vi "Post-Processing VI Bin Files SubSample Tianyi.vi"() -> ()   [LabVIEW 2014]
uses:
  <vilib>/Utility/config.llb/NI_LVConfig.lvlib
  <vilib>/Utility/config.llb/Read Key (I32).vi
  <vilib>/Utility/config.llb/Read Key (Double).vi
  Classes/Processing/Processing.lvclass
panel:
  in  "A-Scan Change":i32=627
  out "BScan":u8[][](graph)
  out "Range":dbl=4.0
  out "Bits":dbl=16.0
  out "Points Per A Scan":i32=1600
  out "A-Scans Per BScan":i32=1000
  in  "Min / Max in dB (Contrast)":cluster{dbl, dbl}(slide)={-34.05144694533762, 14.823151125401928} scale=-40.0..60.0
  in  "Create 3D Data":bool=TRUE
  in  "Max":sgl=14.823152 format="%0.2f"
  in  "Min":sgl=-34.05145 format="%0.2f"
  out "Binary File Handle":refnum<file>
  in  "Create En Face Software Event":bool=TRUE
  out "En Face":sgl[][](graph)=[[-7.930091, -7.8040323, -7.973442, -8.000936, -7.8626037, -7.893125, -7.976362, -7.866958, -7.8874545, -8.053767, -7.895429, -8.001336, -8.058077, -7.9112062, -7.757364, -7.965038, -7.9575043, -8.167074, -8.054711, -8.167959, -7.8551683, -7.915979, -7.9114604, -7.864061, -8.055119, -7.9877367, -8.029805, -7.988413, -8.037094, -7.922483, -8.156847, -7.9672847, -7.8064103, -7.9114566, -7.773133, -7.9002914, -8.085471, -7.9221673, -7.957444, -7.958286, -7.698463, -8.002342, -7.989561, -7.952671, -7.984078, -7.836235, -8.0634165, -8.028308, -8.039231, -8.056543, -7.8877096, -7.9473996, -7.865986, -7.929803, -7.9396944, -7.8729186, -7.962053, -7.976538, -7.829268, -7.759593, -7.6770754, -7.917806, -7.978408, -7.7964263, -7.9014854, -7.8359327, -8.019228, -7.9651647, -7.961875, -8.0167675, -7.915086, -7.975068, -8.046566, -7.960596, -7.990237, -8.160412, -8.09407, -7.795923, -7.8977365, -7.917423, -8.06519, -7.941408, -8.036876, -7.946509, -8.009643, -7.7677317, -8.056414, -8.105821, -8.020063, -7.946077, -7.9010644, -8.056617, -8.010448, -8.0648775, -7.9236917, -7.8220835, -7.8197546, -7.8338175, -7.908895, -7.9036684, -7.9667068, -8.103706, -7.9954534, -7.9504957, -7.829475, -7.831149, -8.244316, -8.030985, -8.157568, -7.6754923, -7.9325967, -8.037667, -7.9114547, -7.946226, -7.8830395, -7.788606, -8.123245, -7.848808, -8.020647, -7.825039, -8.136002, -7.8881106, -7.840354, -7.8498588, -7.868983, -8.012706, -8.025735, -8.1118145, -7.816016, -7.8430986, -7.9750667, -8.042043, -7.820652, -7.8192554, -7.888372, -8.02898, -7.891756, -7.86369, -7.979582, -7.7987456, -8.169637, -7.8604546, -8.097469, -7.882909, -7.745224, -7.9409885, -8.008719, -7.874554, -7.934384, -7.889922, -7.9307194, -7.976539, -7.8116565, -8.037268, -7.8819757, -7.90127, -8.004612, -7.9514766, -7.6461873, -8.051855, -8.033362, -7.820009, -8.007025, -7.9113975, -7.972308, -8.075444, -7.9308887, -8.089264, -7.8016825, -7.919436, -7.94926, -7.7312274, -8.1581135, -7.806207, -7.956523, -7.9414477, -7.9876857, -7.9657526, -7.8116117, -7.8548036, -7.9839373, -7.9158034, -7.898539, -7.780124, -7.9533, -7.8764243, -7.739191, -7.80521, -8.063391, -7.9777446, -7.7854123, -7.9521074, -7.98957, -7.888753, -7.7991505, -7.9267855, -7.9612865, -7.819488, -7.865055, -8.14359, -7.7728977, -8.085733, -7.8384624, -7.743552, -7.886237, -7.9267993, -7.9535413, -7.8223243, -7.8396297, -7.870655, -8.026216, -7.7772164, -7.80645, -8.013777, -8.012371, -7.7353735, -7.935509, -7.860224, -7.9132657, -7.845752, -7.7870827, -7.958748, -8.160488, -7.869349, -7.78722, -7.955144, -7.8493533, -7.8096776, -7.986651, -7.945869, -7.935255, -8.144389, -7.9736667, -7.752922, -7.9255905, -7.974105, -7.799902, -7.6951523, -7.799085, -7.9162817, -8.017551, -7.9524965, -7.9512806, -8.165993, -7.7668185, -8.012505, -8.16206, -8.251981, -8.013035, -7.735666, -8.077859, -8.10991, -7.949526, -7.707088, -7.949591, -7.8823195, -7.816381, -8.034339, -7.868784, -7.89056, -7.8687153, -8.057175, -7.9518924, -7.9154468, -7.939955, -7.814576, -8.049959, -7.9097743, -7.863441, -7.846818, -7.96588, -7.789853, -8.094775, -7.7202816, -8.046873, -8.085813, -7.9780364, -7.9041257, -7.926487, -7.9343805, -8.040627, -7.830686, -8.070694, -7.8358226, -7.7780213, -7.8480616, -8.064976, -8.037013, -7.7728744, -8.012946, -7.9755006, -7.906261, -8.043798, -7.911961, -7.992775, -8.001271, -7.9195423, -8.082046, -8.020159, -7.9112606, -7.775108, -8.003549, -7.9803247, -7.8879714, -8.073655, -7.8865504, -7.783486, -7.8546762, -8.020269, -8.023449, -8.067884, -7.7598515, -7.90917, -8.069023, -7.7864647, -7.870191, -7.870761, -7.9444532, -7.993182, -7.917858, -8.03805, -7.93978, -7.7982545, -7.974645, -8.004379, -7.993704, -7.819672, -8.089255, -7.9242916, -7.907874, -7.9370337, -7.863256, -7.7989616, -7.80284, -8.006147, -7.823976, -7.995604, -8.050512, -7.964656, -8.11802, -7.9949827, -7.951066, -7.7912025, -7.927686, -8.008126, -7.891107, -8.10944, -8.134752, -7.8064127, -7.910995, -8.09849, -7.8788795, -8.016058, -7.8636923, -7.9307437, -7.974993, -7.991549, -7.974662, -7.93784, -7.7311897, -8.182317, -7.7587895, -8.095182, -7.874478, -7.813459, -7.879261, -7.829288, -8.035134, -7.861396, -7.986878, -7.782207, -7.79948, -7.9310637, -7.852276, -7.9916263, -7.9213424, -8.203527, -7.921085, -8.025147, -7.8967156, -7.8208995, -7.9961405, -8.083003, -7.98257, -7.9804964, -7.8674, -8.060883, -7.9558725, -7.945471, -8.142715, -8.087639, -8.218578, -8.243896, -7.959839, -7.9356184, -7.7503934, -8.0898695, -7.868658, -7.692663, -7.887905, -7.8621182, -7.9225054, -7.836562, -8.054047, -7.982782, -7.744281, -7.963519, -8.0447, -7.849429, -7.838456, -8.119481, -7.7900977, -7.9761267, -7.8695583, -7.76462, -7.970638, -7.9605556, -7.964503, -7.9509263, -7.86703, -8.055239, -7.884155, -7.844713, -7.856759, -7.9913874, -8.0371475, -7.938692, -8.049144, -8.021844, -7.7414804, -7.920646, -8.197608, -7.880194, -7.9744005, -8.035382, -8.069501, -8.181021, -8.0188465, -8.004074, -8.031586, -8.0189085, -8.058473, -7.9364552, -7.719303, -7.905371, -7.790757, -8.214631, -7.9018154, -7.987326, -7.9526286, -7.8612223, -7.9100804, -8.08193, -7.9836636, -8.027385, -8.095275, -7.9418774, -7.9966297, -7.9296713, -8.01897, -7.9224367, -7.8740377, -7.8067255, -8.113648, -7.965984, -7.919392, -7.9538283, -7.9669385, -7.9489245, -7.9807835, -8.049196, -8.2190485, -7.967722, -8.009465, -7.814837, -7.9246864, -7.923164, -7.990351, -7.917373, -8.095252, -8.055175, -8.003493, -7.828865, -7.96325, -7.9371457, -7.87614, -7.833712, -8.081883, -7.9843564, -7.8006735, -7.917411, -7.8912277, -7.9116125, -8.126464, -7.9357214, -7.9421554, -7.757199, -7.938931, -7.852307, -8.009288, -7.8433046, -7.8127127, -7.774231, -7.958359, -7.8807616, -8.237229, -8.159578, -7.96494, -8.140689, -7.666607, -7.9215274, -7.7746763, -7.9678416, -8.0088625, -7.897964, -7.9378257, -8.099062, -8.039701, -7.9717793, -8.185365, -8.0567465, -7.9489536, -7.8975363, -8.023378, -7.8149986, -7.7747483, -8.115946, -8.063846, -7.8867245, -7.9420667, -7.8944864, -8.023156, -7.8669634, -7.876997, -7.841495, -7.9707136, -7.9111295, -7.863631, -8.016624, -7.956105, -7.858278, -8.059558, -8.096037, -7.892564, -7.9129233, -7.79077, -7.9832497, -7.985417, -7.7849727, -8.001589, -7.7398777, -7.7428336, -7.906874, -8.126725, -8.015352, -8.038417, -7.965966, -7.911179, -7.9052196, -7.9147563, -7.75231, -8.021024, -7.8436966, -8.057442, -7.9307613, -7.822249, -8.146226, -8.007187, -7.6794977, -7.83178, -7.8921013, -8.013386, -8.003119, -7.9583955, -7.938617, -8.110327, -8.210196, -7.9229064, -7.970181, -7.8199425, -8.0372505, -7.8034477, -7.8715796, -8.105112, -7.8673153, -7.9806876, -7.944533, -7.8558373, -8.031324, -8.0394125, -7.9362345, -7.8742948, -8.004431, -7.9117155, -7.92383, -8.22453, -7.9384084, -8.046981, -7.948592, -7.9943843, -8.039814, -7.867514, -7.8567586, -7.7503667, -8.132967, -7.8055544, -8.099513, -8.015846, -7.80609, -8.167438, -7.801515, -7.9792643, -7.9695144, -7.709452, -7.8683558, -7.7977037, -7.904273, -7.790883, -8.073817, -8.044217, -7.6886067, -7.854426, -7.841001, -7.8545475, -8.139268, -7.948963, -7.89186, -7.8355184, -7.917378, -7.9529567, -7.8986993, -7.7398877, -7.946703, -7.9786987, -8.031789, -7.9741163, -7.870274, -7.9702334, -8.02977, -7.8809557, -7.8097644, -7.9288607, -8.126841, -7.8123865, -7.8626604, -7.8187237, -7.8525906, -7.9653254, -7.9950914, -7.9080153, -8.03097, -7.805545, -7.777243, -7.77037, -8.001218, -8.017348, -8.007549, -7.8903728, -7.851192, -7.73721, -7.894369, -7.9804764, -7.972263, -8.017426, -7.9188137, -7.699553, -7.985173, -8.14926, -7.9460635, -7.9795494, -8.0467, -7.855538, -7.912811, -7.9511986, -7.9749317, -7.9023323, -7.9952846, -7.9592586, -8.030751, -7.920987, -7.924575, -7.641929, -7.819344, -7.847093, -7.996105, -7.60953, -7.8648734, -8.019921, -7.804081, -7.8468595, -7.806482, -7.854887, -7.9134655, -7.771183, -7.8451014, -8.077572, -8.037743, -7.8422785, -8.027252, -7.953315, -7.8755074, -7.9896126, -7.8166866, -8.076665, -7.956374, -8.030051, -7.9240355, -7.884757, -7.8483443, -7.8289475, -8.139085, -7.770633, -7.9318833, -8.016564, -7.8698854, -7.7932873, -7.8172855, -7.8905444, -7.986914, -7.9401693, -7.9614263, -7.9716263, -7.9189005, -8.085335, -7.7258472, -8.012342, -7.7290063, -7.962374, -7.736857, -7.908464, -7.95836, -7.727169, -7.9340315, -8.031877, -7.887279, -7.8412385, -8.041202, -7.8045454, -7.8905506, -7.7506995, -7.9316373, -7.9499393, -7.851978, -7.9120736, -7.9021235, -7.8550596, -7.8048263, -7.946267, -8.050364, -7.9034224, -7.9725904, -7.869547, -7.885991, -7.968221, -7.78149, -7.824945, -7.8112597, -7.997913, -8.123039, -7.8428135, -8.064973, -7.86549, -7.898531, -7.871154, -7.8630815, -8.026972, -8.056086, -8.107686, -7.9592414, -7.802565, -7.8990717, -7.8917937, -7.9946303, -7.935857, -7.7870903, -7.925476, -8.08807, -7.9506598, -7.903563, -7.7953897, -7.938492, -7.7871675, -7.921679, -7.8528447, -8.03581, -7.8427415, -7.889442, -7.972731, -8.008952, -7.9870386, -7.81934, -8.098788, -7.990713, -7.902563, -8.00334, -8.157312, -7.8009663, -7.755303, -8.165585, -8.05285, -7.908865, -7.8209777, -7.978314, -7.8780475, -7.93847, -7.8299446, -7.8623195, -7.93139, -7.7586055, -7.9444237, -7.8643084, -7.877962, -8.007582, -7.7742763, -7.890612, -8.051581, -7.892482, -7.8677154, -7.927973, -7.8819814, -7.9347353, -7.999919, -8.090686, -7.8633533, -7.88977, -8.057978, -8.034815, -7.7877083, -7.817199, -7.9679923, -8.017427, -7.9522886, -7.943636, -7.9850945, -7.99855, -7.863006, -7.88045, -8.068299, -7.925362, -8.142173, -7.8893266, -7.957223, -7.7491736, -7.852534, -8.071495, -7.865574, -7.799149, -7.8367667, -7.996641, -8.050482, -8.003815, -7.783416, -8.051039, -7.9302397, -8.008375, -7.833727, -7.8489013, -7.9530954, -7.9982214, -7.953154, -7.9360614, -8.100909, -7.979594, -7.670946, -8.022225, -7.8406134, -8.0095, -8.040179, -7.865175, -7.9610953, -8.07941, -7.9528823, -7.8656754, -7.979678, -7.802908, -7.972213, -7.9385486, -8.097144, -7.7224145, -7.8400908, -7.9734745, -8.105193, -7.8446107, -7.968687, -7.7581, -8.128169, -8.130323, -7.7925196, -8.015969, -7.678966, -7.872306, -7.836657, -7.9079814, -7.84879, -8.133352, -7.889341, -8.066047, -7.982547, -7.951533, -7.902655, -8.105811, -7.97907, -7.9479356, -7.960124, -7.8474517, -8.111724, -7.9724307, -7.975754, -7.985938, -7.9817557, -7.78798, -8.040827, -7.760837, -7.8727965, -7.984424, -8.078643, -7.885198, -7.9081254, -7.7833333, -7.908534, -7.6961055, -7.913281, -7.7185884, -8.042309, -8.115078, -8.14631, -7.806838, -7.7963495, -8.055587, -7.97538, -7.698462, -7.775273, -8.045425, -8.037591, -8.0973015, -7.7711625, -7.988266, -7.9091988, -7.8253546, -7.925254, -7.9461355, -7.766041, -7.8593016, -7.9350066, -8.008051, -7.861942, -7.8998094, -8.016808, -8.124489, -7.9874635, -8.083402, -8.1051035, -7.993055, -7.880184, -7.91285, -7.9538074, -7.9280205, -8.043174, -8.137445, -8.110672, -7.897486, -7.9666576, -7.978455, -7.9780507, -8.032585, -8.116778, -7.971109, -7.824977, -7.766515, -7.981128, -7.930899, -8.109892, -7.9214025, -7.8610687, -7.839897, -8.006488, -7.792739, -7.9065375, -8.032204, -7.81708, -7.790314, -8.064906, -8.093157, -7.839383, -8.11415, -7.9893, -8.070883, -8.176108, -7.7919936, -8.105036, -8.017701, -8.068903, -8.093538, -7.8479977, -7.9812527, -7.871276, -7.8107314, -7.958203, -7.8588, -7.829434]]
  out "error out":errorcluster
  in  "En Face Upper Depth":i32=60
  in  "En Face Lower Depth":i32=300
  in  "B-Scan Select":i32(slide) scale=0.0..128.0
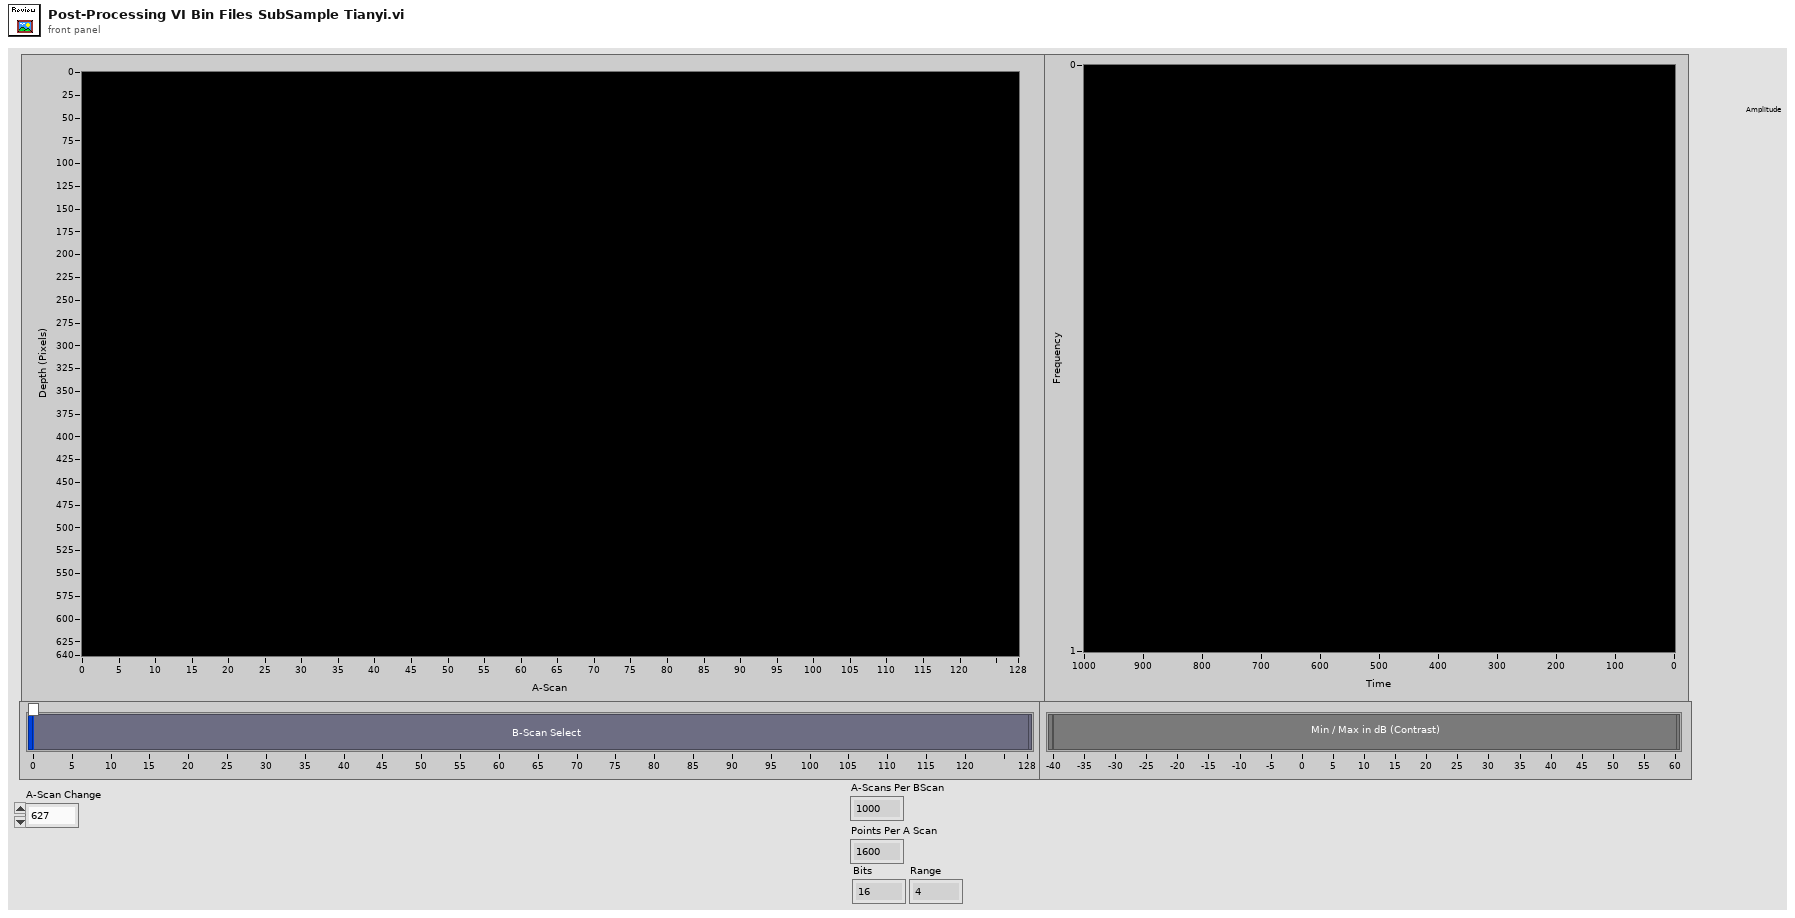
[diagram p1: front panel]
types:
  T1 = enum32{"Invalid", "Standard", "Closed", "Hidden", "Minimized", "Maximized"}
  T2 = typedef "NI_LVConfig.lvlib/Config Data RefNum.ctl" = refnum<k1>
  T3 = typedef "imagedata.ctl" = cluster{"image type":i32, "image depth":i32, "image":u8[], "mask":u8[], "colors":u32[], "Rectangle":cluster{"left":i16, "top":i16, "right":i16, "bottom":i16}}
  T4 = typedef "LVCursorListTypeDef.ctl" = cluster{"Name":string, "Color":u32, "Style":u8, "Point Style":u8, "Name Visible":bool, "Allow Drag":bool, "Cursor Mode":u32, "Plot":i32, "Index":i32, "Position":cluster{"X":dbl, "Y":dbl}, "X Scale":u32, "Y Scale":u32, "Watch Plots":i32[], "Watch All Plots":bool, "Plot Area":i32, "Label Offset":cluster{"X":dbl, "Y":dbl}}[]
  T5 = cluster{"Name":string, "Color":u32, "Style":u8, "Point Style":u8, "Name Visible":bool, "Allow Drag":bool, "Cursor Mode":u32, "Plot":i32, "Index":i32, "Position":cluster{"X":dbl, "Y":dbl}, "X Scale":u32, "Y Scale":u32, "Watch Plots":i32[], "Watch All Plots":bool, "Plot Area":i32, "Label Offset":cluster{"X":dbl, "Y":dbl}}
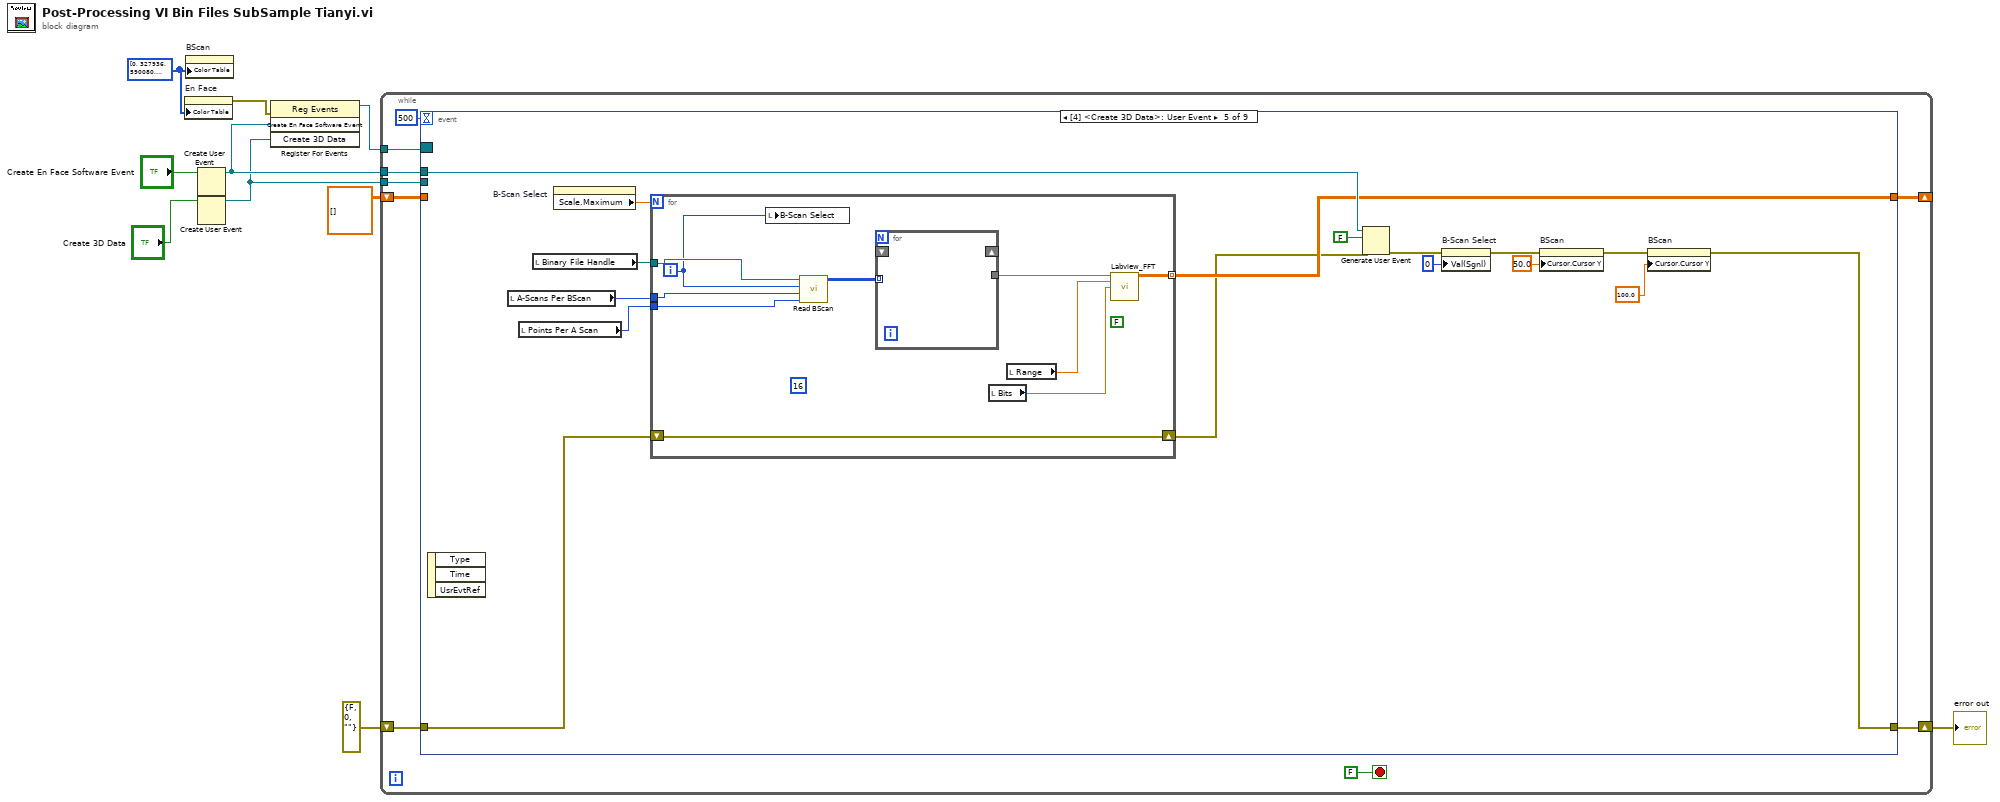
[diagram p0: block diagram]
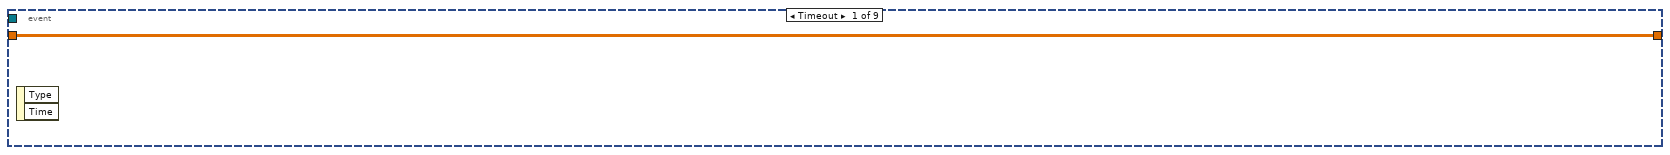
[diagram p2: hidden frame]
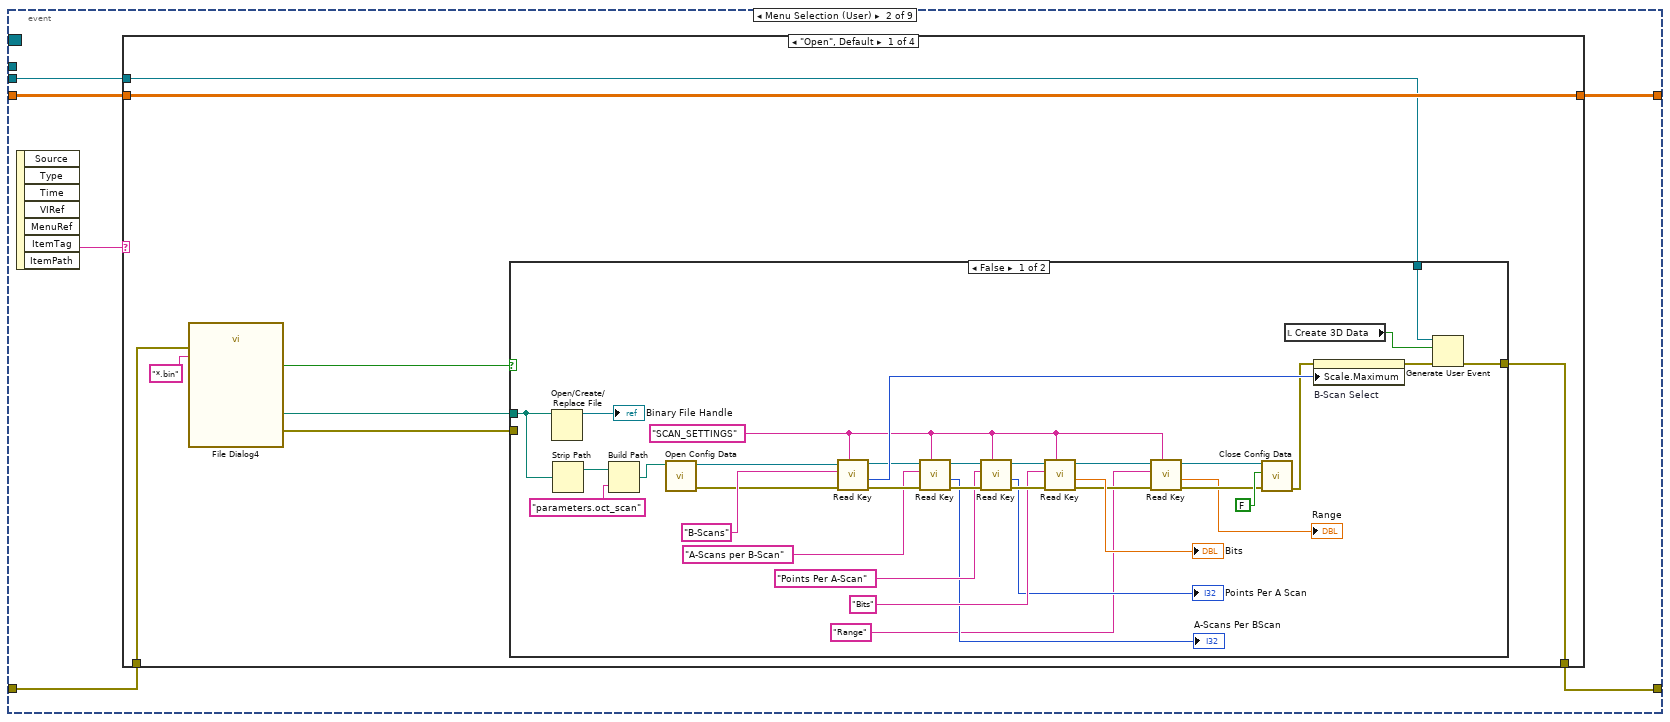
[diagram p3: hidden frame]
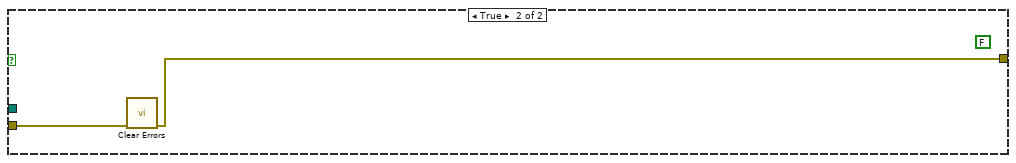
[diagram p4: hidden frame]
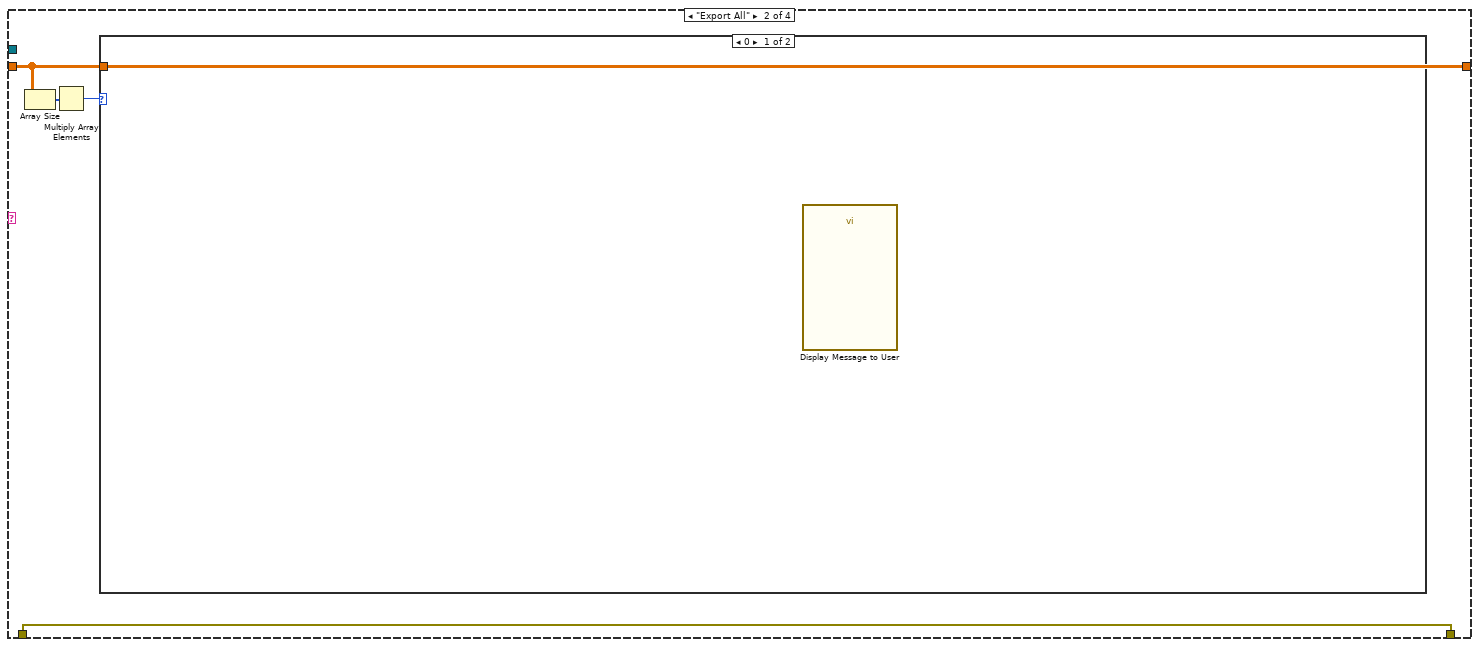
[diagram p5: hidden frame]
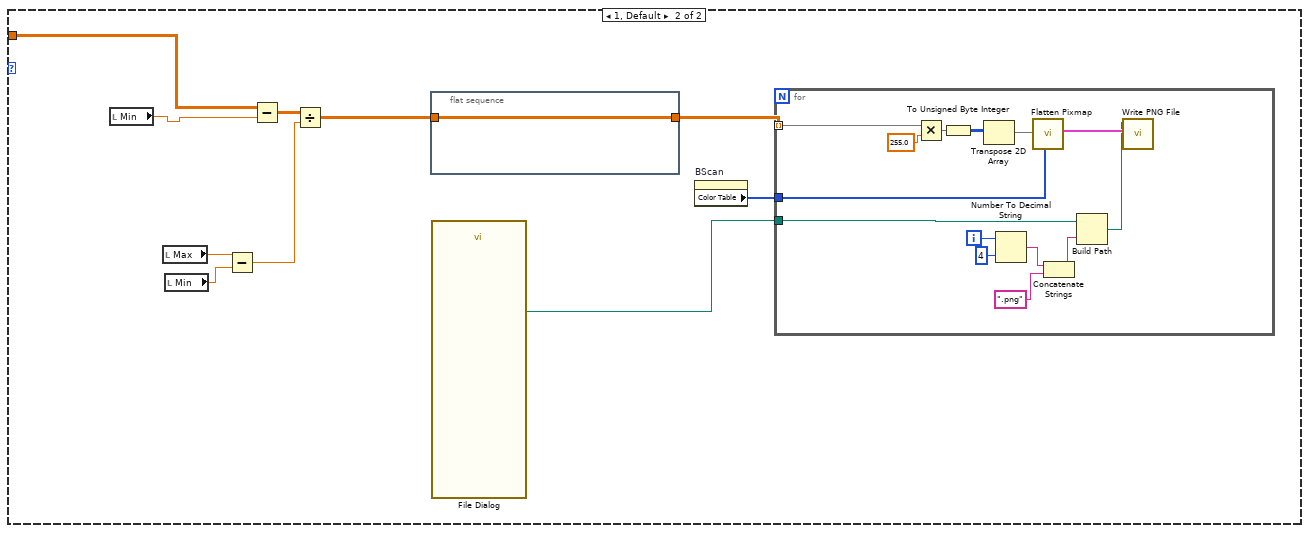
[diagram p6: hidden frame]
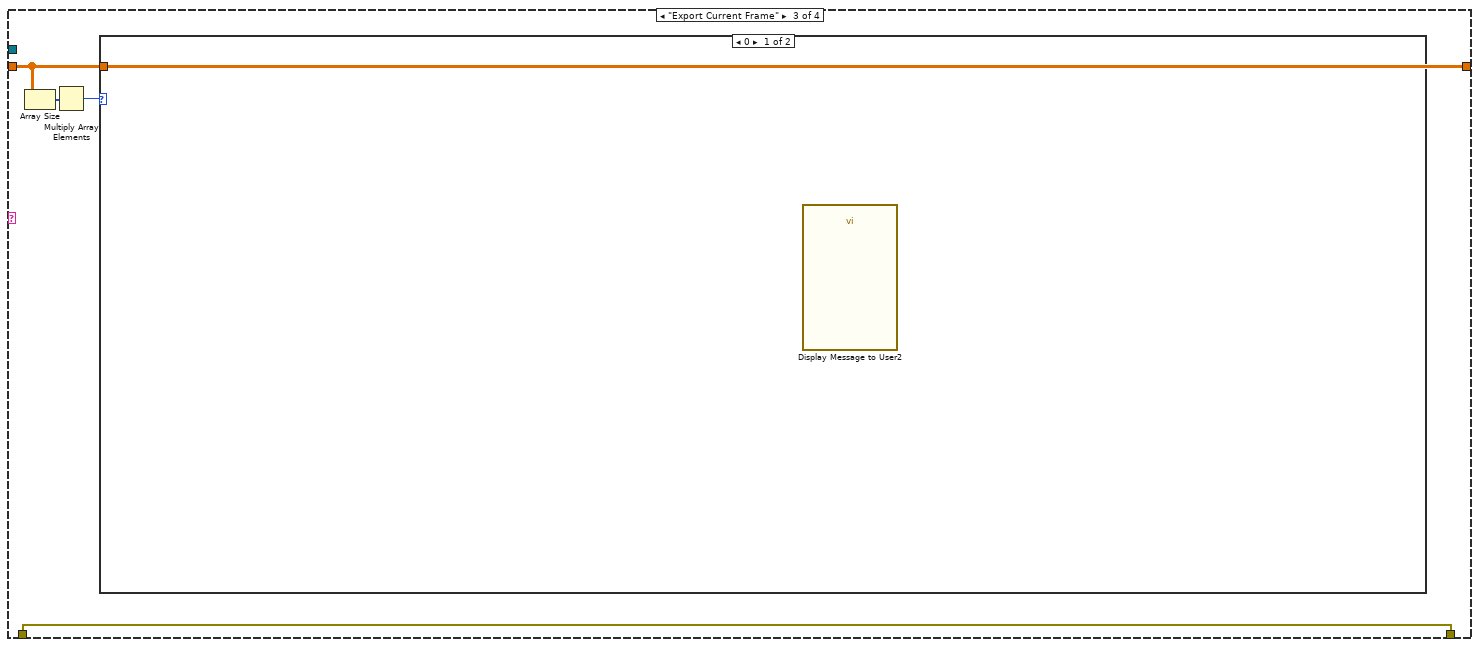
[diagram p7: hidden frame]
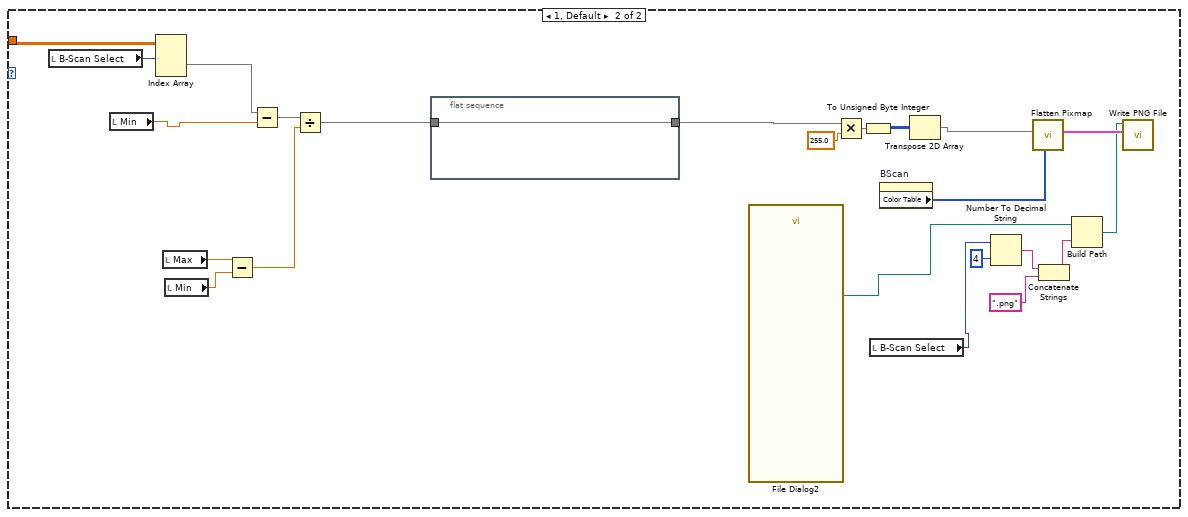
[diagram p8: hidden frame]
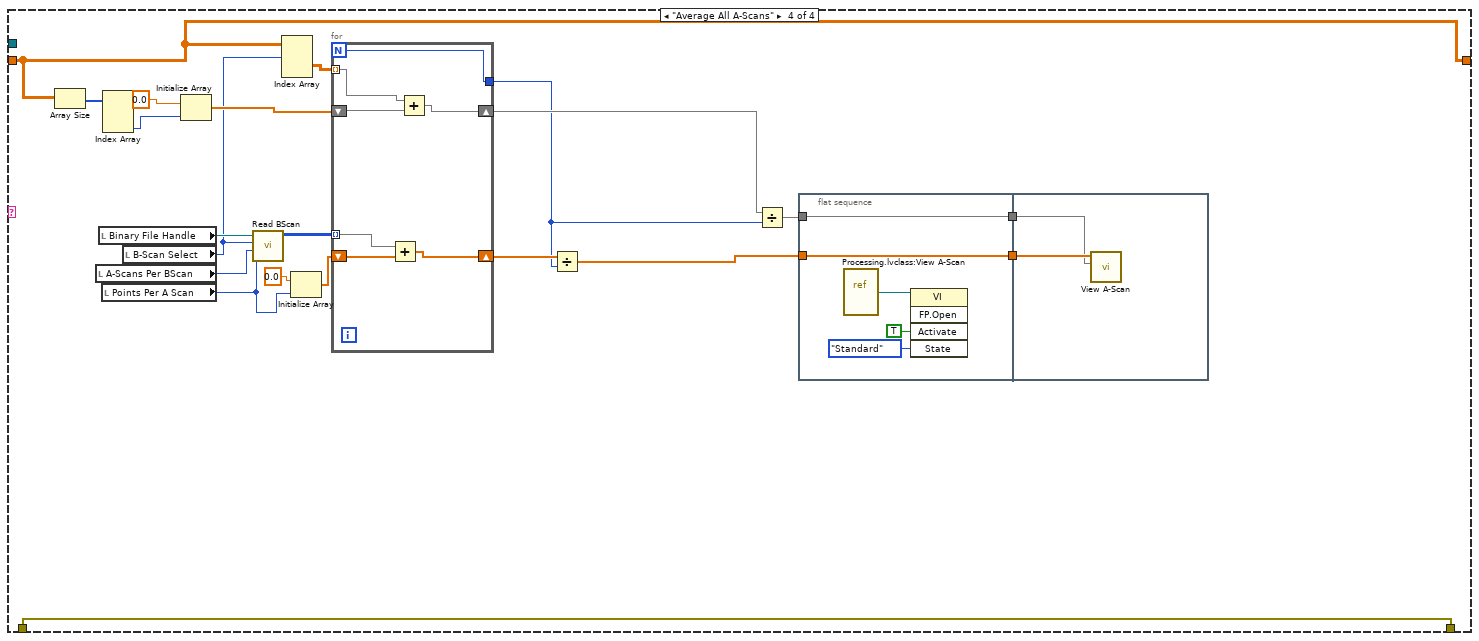
[diagram p9: hidden frame]
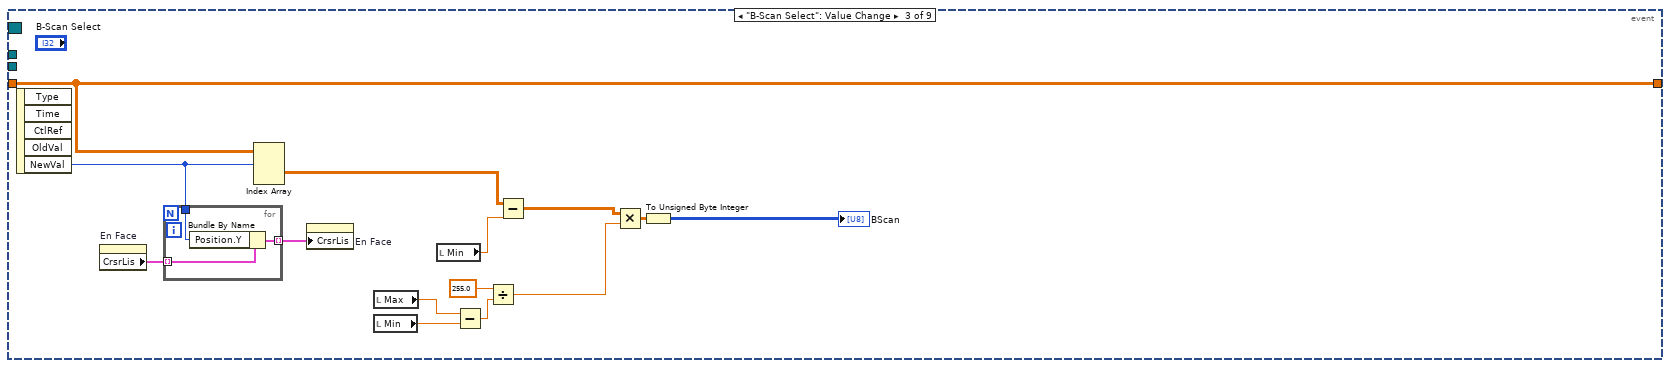
[diagram p10: hidden frame]
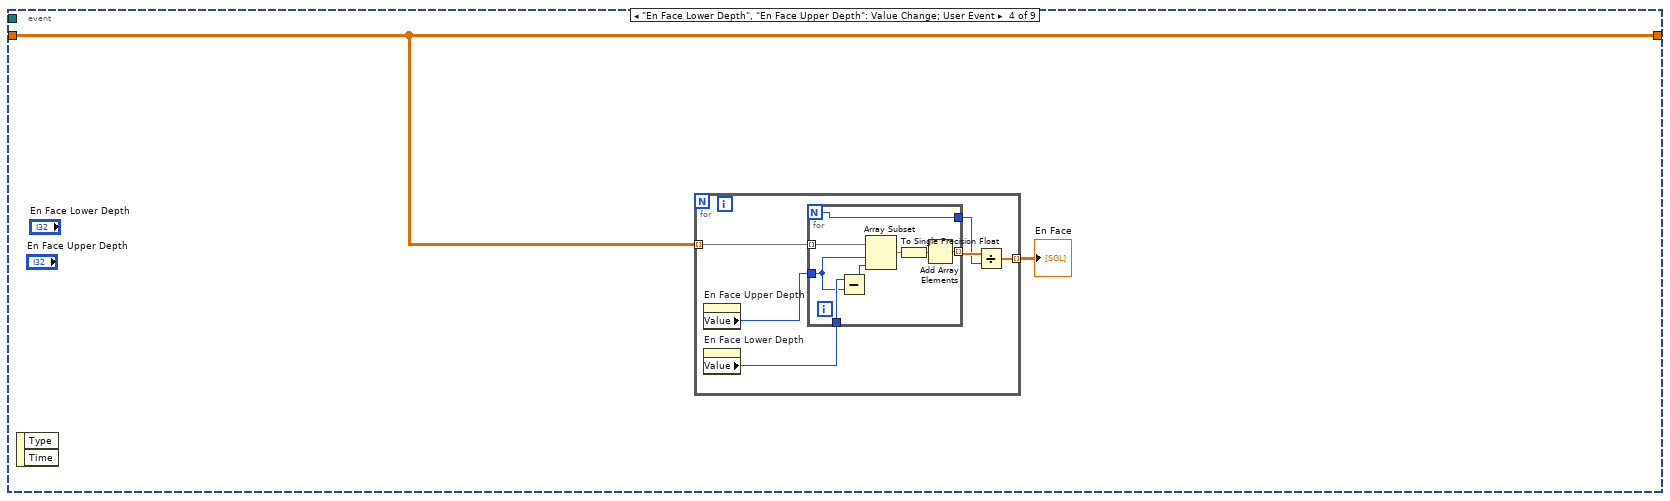
[diagram p11: hidden frame]
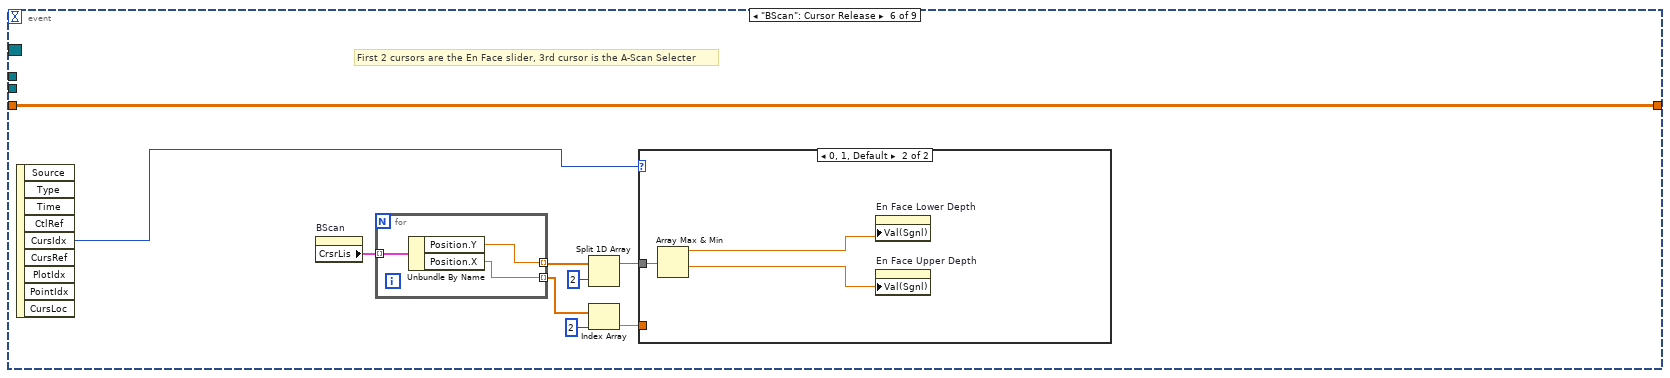
[diagram p12: hidden frame]
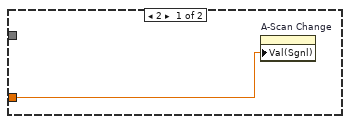
[diagram p13: hidden frame]
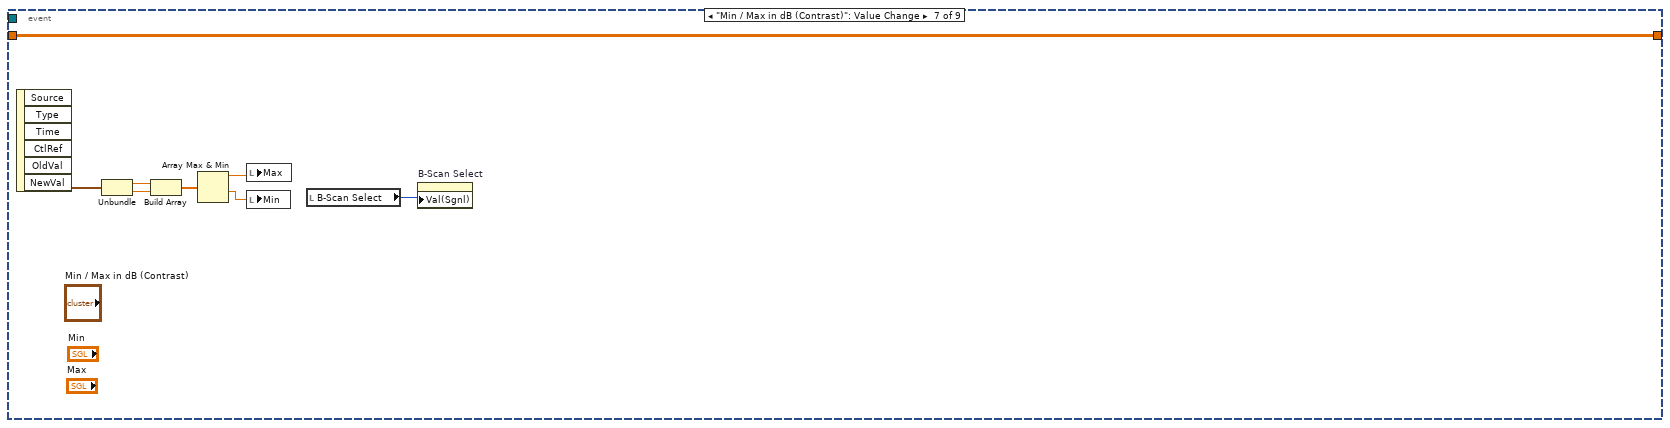
[diagram p14: hidden frame]
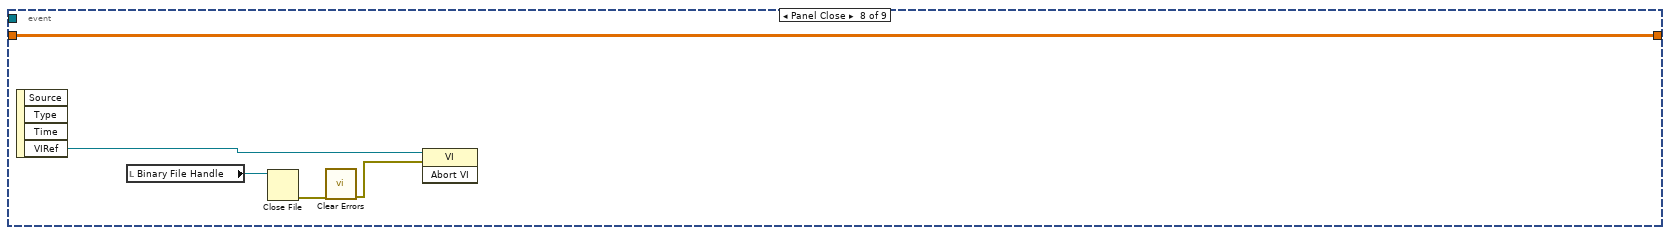
[diagram p15: hidden frame]
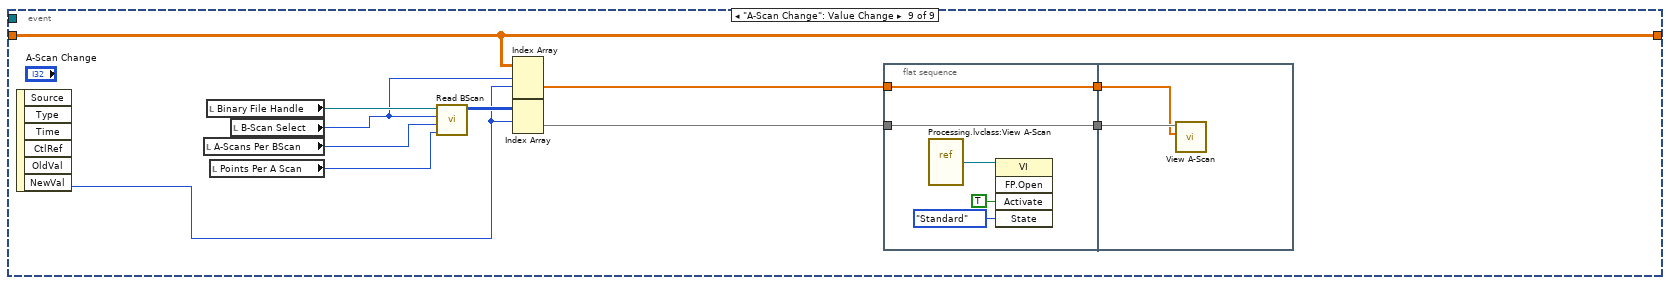
[diagram p16: hidden frame]
diagram:
  w3 = u32[] [0, 327936, 590080, 852224, 983296, 1114624, 1180160, 1311232, 1442304, 1573632, 1704704, 1770240, 1901312, 1966848, 2098176, 2163712, 2294784, 2491392, 2557184, 2688256, 2753792, 2884864, 2950656, 3081728, 3147264, 3344129, 3475457, 3540993, 3672321, 3738113, 3869185, 3934977, 4066305, 4197633, 4328961, 4394497, 4460289, 4591617, 4657409, 4788481, 4854273, 4985601, 5116929, 5248257, 5314049, 5379841, 5511169, 5576961, 5708033, 5773825, 5905153, 6036482, 6167810, 6233346, 6299138, 6430466, 6496258, 6562050, 6693634, 6759426, 6890754, 7022082, 7087874, 7153666, 7284994, 7350786, 7482114, 7547906, 7613698, 7745026, 7876354, 8007682, 8073474, 8139522, 8205314, 8336642, 8467970, 8533763, 8599555, 8665347, 8731139, 8862467, 8993795, 9059587, 9125380, 9191428, 9257220, 9388548, 9454340, 9520132, 9585924, 9717253, 9848837, 9914629, 9980165, 10045957, 10177541, 10243334, 10309126, 10375174, 10440966, 10572294, 10703623, 10769416, 10835208, 10901256, 10967049, 11033097, 11033609, 11099401, 11165450, 11231242, 11231754, 11297547, 11363339, 11429131, 11495180, 11495692, 11561740, 11693069, 11758861, 11759373, 11825165, 11891214, 11957006, 12022799, 12023311, 12089103, 12220944, 12286736, 12286736, 12352529, 12418577, 12484370, 12550162, 12615954, 12681747, 12747796, 12813588, 12813845, 12879894, 12945686, 13077015, 13142808, 13143064, 13208856, 13274905, 13340697, 13340953, 13472282, 13538075, 13604379, 13670172, 13735964, 13801757, 13867550, 13933343, 13999392, 13999648, 14065441, 14131234, 14197027, 14197541, 14263334, 14329383, 14395176, 14460969, 14592553, 14658346, 14724139, 14789932, 14790189, 14856238, 14922287, 14988080, 15053873, 15054130, 15119923, 15185972, 15251765, 15317559, 15383353, 15449146, 15449660, 15515454, 15515968, 15516226, 15582021, 15582278, 15582536, 15648587, 15648844, 15714639, 15714897, 15715155, 15780949, 15781463, 15847256, 15847770, 15848028, 15913823, 15914081, 15979875, 15980133, 15980391, 16046441, 16046444, 16046703, 16046705, 16112500, 16113015, 16113274, 16113277, 16179072, 16179330, 16179588, 16245384, 16245387, 16245389, 16245648, 16311443, 16376982, 16377241, 16377499, 16443294, 16443553, 16443555, 16443815, 16509866, 16510124, 16510127, 16575923, 16575924, 16576182, 16576441, 16576443, 16576702, 16576705, 16576963, 16577222, 16577224, 16577482, 16577485, 16577743, 16577745, 16578004, 16578262, 16578264, 16578523, 16578782, 16579040, 16579299, 16579301, 16579303, 16579562, 16579821] ("Color Table")
  n1 = property on="En Face" class="IntGraph (strict)"("Color Table"=w3) -> (error out=w2:errorcluster)  [unwired: 2 in, 1 out]
  n2 = property on="BScan" class="IntGraph (strict)"("Color Table"=w3) -> ()  [unwired: 2 in, 2 out]
  n3 = Create User Event(user event datatype="Create En Face Software Event") -> (user event=w9:refnum<user-event>)  [unwired: 1 in, 1 out]
  n4 = Create User Event(user event datatype="Create 3D Data") -> (user event=w8:refnum<user-event>)  [unwired: 1 in, 1 out]
  n5 = register-events(error in=w2, w9, w8) -> (reference out=w10:refnum<event-registration>)  [unwired: 1 in, 1 out]
  n6 = while {
    tunnel: w10 -> [w17]
    tunnel: w9 -> [w16]
    tunnel: w8 -> [w15]
    shift-right: [w13] -> w4
    shift-left: errorcluster {"status"=FALSE, "code"=0, "source"=""} ("error constant") -> [w14]
    shift-right: [w11] -> _
    shift-left: sgl[][][] [] ("Int B-Scan Channel A") -> [w12]
    stop <- FALSE stop-if-true
    n7 = event shown="[4] <Create 3D Data>: User Event" {
      selector: w17 -> [_ _ _ _ _ _ _ _ _]
      dyn-events: _ -> [_ _ _ _ _ _ _ _ _]
      timeout: 500 -> [_ _ _ _ _ _ _ _ _]
      tunnel: w15 -> [_ w23 _ _ _ _ _ _ _]
      tunnel: w16 -> [_ _ _ _ w208 _ _ _ _]
      tunnel: w14 -> [_ w22 _ _ w207 _ _ _ _]
      tunnel: [_ w21 _ _ w199 _ _ _ _] -> w13
      tunnel: w12 -> [w20 w25 w163 w180 _ w230 w238 w249 w257]
      tunnel: [w20 w24 w163 w180 w204 w230 w238 w249 w257] -> w11
      event Timeout {
        n8 = event-data() -> ()  [unwired: 1 in, 2 out]
      }
      event Menu Selection (User) {
        n9 = event-data() -> ("ItemTag"=w26:string)  [unwired: 1 in, 6 out]
        n10 = case shown="\"Open\", Default" w26 {
          tunnel: w25 -> [w34 w73 w102 w141]
          tunnel: [w34 w73 w102 w141] -> w24
          tunnel: w23 -> [w28 _ _ _]
          tunnel: w22 -> [w31 w74 w103 w148]
          tunnel: [w27 w74 w103 w148] -> w21
          frame "Open", Default {
            n11 = call "File Dialog4"("error in"=w31, "pattern (all files)"="*.bin") -> ("selected path"=w32:path, "cancelled"=w30:bool, "error out"=w29:errorcluster)  [unwired: 10 in, 1 out]
            n12 = case shown="False" w30 {
              tunnel: [w37 w69] -> w27
              tunnel: w32 -> [w67 _]
              tunnel: w29 -> [_ w70]
              tunnel: w28 -> [w36 _]
              frame False {
                w43 = "SCAN_SETTINGS" ("section")
                n13 = Open/Create/Replace File(file path (use dialog)=w67) -> (refnum out=→"Binary File Handle":refnum<file>)  [unwired: 5 in, 2 out]
                n14 = Strip Path(path=w67) -> (stripped path=w66:path)  [unwired: 1 out]
                n15 = Build Path(base path=w66, name or relative path="parameters.oct_scan") -> (appended path=w64:path)
                n16 = call <vilib>:"Open Config Data.vi"("configuration file path"=w64) -> ("error out"=w62:errorcluster, "refnum"=w61:T2)  [unwired: 8 in, 1 out]
                n17 = call-poly <vilib>:"Read Key.vi"("section"=w43, "error in (no error)"=w62, "key"="B-Scans", "refnum"=w61) -> ("error out"=w58:errorcluster, "value"=w60:i32, "refnum out"=w57:T2)  [unwired: 4 in, 1 out]
                n18 = call-poly <vilib>:"Read Key.vi"("section"=w43, "error in (no error)"=w58, "key"="A-Scans per B-Scan", "refnum"=w57) -> ("error out"=w55:errorcluster, "value"=→"A-Scans Per BScan":i32, "refnum out"=w54:T2)  [unwired: 4 in, 1 out]
                n19 = call-poly <vilib>:"Read Key.vi"("section"=w43, "error in (no error)"=w55, "key"="Points Per A-Scan", "refnum"=w54) -> ("error out"=w52:errorcluster, "value"=→"Points Per A Scan":i32, "refnum out"=w51:T2)  [unwired: 4 in, 1 out]
                n20 = call-poly <vilib>:"Read Key.vi"("section"=w43, "error in (no error)"=w52, "key"="Bits", "refnum"=w51) -> ("error out"=w44:errorcluster, "value"=→"Bits":dbl, "refnum out"=w45:T2)  [unwired: 4 in, 1 out]
                n21 = call-poly <vilib>:"Read Key.vi"("section"=w43, "error in (no error)"=w44, "key"="Range", "refnum"=w45) -> ("error out"=w40:errorcluster, "value"=→"Range":dbl, "refnum out"=w41:T2)  [unwired: 4 in, 1 out]
                n22 = call <vilib>:"Close Config Data.vi"("error in (no error)"=w40, "write file if changed (T)"=FALSE, "refnum"=w41) -> ("error out"=w49:errorcluster)  [unwired: 7 in, 1 out]
                n23 = local read "Create 3D Data"() -> (w35:bool)
                n24 = property on="B-Scan Select" class="Slide (strict)"(error in=w49, "Scale.Maximum"=w60) -> (error out=w38:errorcluster)  [unwired: 1 in, 1 out]
                n25 = Generate User Event(user event=w36, event data cluster=w35, error in=w38) -> (error out=w37:errorcluster)  [unwired: 1 in, 1 out]
              }
              frame True {
                (unwired) FALSE ("Create 3D Data")
                n26 = call <vilib>:"Clear Errors.vi"("error in (no error)"=w70) -> ("error out"=w69:errorcluster)  [unwired: 5 in, 1 out]
              }
            }
          }
          frame "Export All" {
            n27 = Array Size(array=w73) -> (size(s)=w72:i32[])
            n28 = Multiply Array Elements(1:w72) -> (0:w71:i32)
            n29 = case shown="0" w71 {
              tunnel: w73 -> [_ w84]
              frame 0 {
                n30 = call "Display Message to User"() -> ()  [unwired: 10 in, 2 out]
              }
              frame 1, Default {
                n31 = local read "Min"() -> (w78:sgl)
                n32 = local read "Max"() -> (w77:sgl)
                n33 = local read "Min"() -> (w76:sgl)
                n34 = Subtract(x=w77, y=w76) -> (x-y=w82:sgl)
                n35 = Subtract(x=w84, y=w78) -> (x-y=w83:sgl[][][])
                n36 = Divide(x=w83, y=w82) -> (x/y=w81:sgl[][][])
                n37 = flat-sequence {
                  tunnel: [w99] -> w80
                  tunnel: w81 -> [w99]
                  frame #0 {
                  }
                }
                n38 = call "File Dialog"() -> ("selected path"=w79:path)  [unwired: 12 in, 3 out]
                n39 = property on="BScan" class="IntGraph (strict)"() -> ("Color Table"=w75:u32[])  [unwired: 2 in, 2 out]
                n40 = for {
                  tunnel: w80 -> [w98] mode=indexing
                  tunnel: w79 -> [w92]
                  tunnel: w75 -> [w85]
                  i -> [w95]
                  n41 = Multiply(x=w98, y=sgl 255.0) -> (x*y=w96:sgl[][])
                  n42 = To Unsigned Byte Integer(number=w96) -> (unsigned 8bit integer=w87:u8[][])
                  n43 = Transpose 2D Array(2D array=w87) -> (transposed array=w86:u8[][])
                  n44 = Number To Decimal String(number=w95, width (-)=i16 4) -> (decimal integer string=w90:string)
                  n45 = call <vilib>:"Flatten Pixmap.vi"("colors"=w85, "8-bit pixmap"=w86) -> ("image data"=w93:T3)  [unwired: 9 in]
                  n46 = Concatenate Strings(w90, ".png" ("string")) -> (w88:string)
                  n47 = Build Path(base path=w92, name or relative path=w88) -> (appended path=w91:path)
                  n48 = call <vilib>:"Write PNG File.vi"("image data"=w93, "path to PNG file"=w91) -> ()  [unwired: 8 in, 2 out]
                }
              }
            }
          }
          frame "Export Current Frame" {
            n49 = Array Size(array=w102) -> (size(s)=w101:i32[])
            n50 = Multiply Array Elements(1:w101) -> (0:w100:i32)
            n51 = case shown="0" w100 {
              tunnel: w102 -> [_ w109]
              frame 0 {
                n52 = call "Display Message to User2"() -> ()  [unwired: 10 in, 2 out]
              }
              frame 1, Default {
                n53 = local read "B-Scan Select"() -> (w110:i32)
                n54 = local read "Min"() -> (w121:sgl)
                n55 = Index Array(array=w109, index (dim 0)=w110) -> (element=w108:sgl[][])  [unwired: 2 in]
                n56 = local read "Max"() -> (w120:sgl)
                n57 = local read "Min"() -> (w119:sgl)
                n58 = Subtract(x=w120, y=w119) -> (x-y=w125:sgl)
                n59 = Subtract(x=w108, y=w121) -> (x-y=w126:sgl[][])
                n60 = Divide(x=w126, y=w125) -> (x/y=w124:sgl[][])
                n61 = flat-sequence {
                  tunnel: [w127] -> w123
                  tunnel: w124 -> [w127]
                  frame #0 {
                  }
                }
                n62 = call "File Dialog2"() -> ("selected path"=w122:path)  [unwired: 12 in, 3 out]
                n63 = Multiply(x=w123, y=sgl 255.0) -> (x*y=w117:sgl[][])
                n64 = To Unsigned Byte Integer(number=w117) -> (unsigned 8bit integer=w105:u8[][])
                n65 = local read "B-Scan Select"() -> (w107:i32)
                n66 = property on="BScan" class="IntGraph (strict)"() -> ("Color Table"=w106:u32[])  [unwired: 2 in, 2 out]
                n67 = Transpose 2D Array(2D array=w105) -> (transposed array=w104:u8[][])
                n68 = Number To Decimal String(number=w107, width (-)=i16 4) -> (decimal integer string=w113:string)
                n69 = call <vilib>:"Flatten Pixmap.vi"("colors"=w106, "8-bit pixmap"=w104) -> ("image data"=w115:T3)  [unwired: 9 in]
                n70 = Concatenate Strings(w113, ".png" ("string")) -> (w111:string)
                n71 = Build Path(base path=w122, name or relative path=w111) -> (appended path=w114:path)
                n72 = call <vilib>:"Write PNG File.vi"("image data"=w115, "path to PNG file"=w114) -> ()  [unwired: 8 in, 2 out]
              }
            }
          }
          frame "Average All A-Scans" {
            n73 = Array Size(array=w141) -> (size(s)=w147:i32[])
            n74 = local read "A-Scans Per BScan"() -> (w143:i32)
            n75 = local read "Binary File Handle"() -> (w144:refnum<file>)
            n76 = local read "Points Per A Scan"() -> (w128:i32)
            n77 = Index Array(array=w147) -> (element #3=w139:i32)  [unwired: 3 in, 2 out]
            n78 = local read "B-Scan Select"() -> (w138:i32)
            n79 = Initialize Array(sgl 0.0 ("element"), w139) -> (w142:sgl[])
            n80 = call "Read BScan.vi"("Points Per A Scan"=w128, "A-Scans Per BScan"=w143, "B-Scan"=w138, "Byte Stream File in"=w144) -> ("Array"=w145:u16[][])  [unwired: 7 in]
            n81 = Index Array(array=w141, index (dim 0)=w138) -> (element=w140:sgl[][])  [unwired: 2 in]
            n82 = Initialize Array(sgl 0.0 ("element"), w128) -> (w130:sgl[])
            n83 = for {
              N -> [w159]
              tunnel: w140 -> [w161] mode=indexing
              shift-right: [w160] -> w132
              shift-left: w142 -> [w162]
              tunnel: [w159] -> w131
              shift-right: [w156] -> w135
              shift-left: w130 -> [w158]
              tunnel: w145 -> [w157] mode=indexing
              n84 = Add(x=w157, y=w158) -> (x+y=w156:sgl[])
              n85 = Add(x=w161, y=w162) -> (x+y=w160:sgl[])
            }
            n86 = Divide(x=w135, y=w131) -> (x/y=w134:sgl[])
            n87 = Divide(x=w132, y=w131) -> (x/y=w133:sgl[])
            n88 = flat-sequence {
              tunnel: w133 -> [w152]
              tunnel: w134 -> [w153]
              tunnel: [w153] -> w137
              tunnel: [w152] -> w136
              tunnel: w137 -> [w155]
              tunnel: w136 -> [w154]
              frame #0 {
                n89 = vi-ref "Processing.lvclass:View A-Scan.vi"() -> (w149:refnum<vi>)
                n90 = invoke class="VI" method="FP.Open"(reference=w149, "Activate"=TRUE ("Activate?"), "State"=T1."Standard") -> ()  [unwired: 2 in, 5 out]
              }
              frame #1 {
                n91 = call "View A-Scan.vi"("A-Scan Processed"=w154, "A-Scan (Raw)"=w155) -> ()  [unwired: 10 in]
              }
            }
          }
        }
      }
      event "B-Scan Select": Value Change {
        n92 = event-data() -> ("NewVal"=w175:i32)  [unwired: 1 in, 4 out]
        n93 = property on="En Face" class="IntGraph (strict)"() -> ("CrsrLis"=w176:T4)  [unwired: 2 in, 2 out]
        n94 = for {
          tunnel: w176 -> [w179] mode=indexing
          tunnel: w175 -> [w178]
          tunnel: [w177] -> w174 mode=indexing
          n95 = Bundle By Name(cluster=w179, "Position.Y"=w178) -> (w177:T5)
        }
        n96 = Index Array(array=w163, index (dim 0)=w175) -> (element=w164:sgl[][])  [unwired: 2 in]
        n97 = property on="En Face" class="IntGraph (strict)"("CrsrLis"=w174) -> ()  [unwired: 2 in, 2 out]
        n98 = local read "Max"() -> (w172:sgl)
        n99 = local read "Min"() -> (w171:sgl)
        n100 = local read "Min"() -> (w166:sgl)
        n101 = Subtract(x=w172, y=w171) -> (x-y=w170:sgl)
        n102 = Divide(x=sgl 255.0, y=w170) -> (x/y=w168:sgl)
        n103 = Subtract(x=w164, y=w166) -> (x-y=w169:sgl[][])
        n104 = Multiply(x=w169, y=w168) -> (x*y=w167:sgl[][])
        n105 = To Unsigned Byte Integer(number=w167) -> (unsigned 8bit integer=→"BScan":u8[][])
      }
      event "En Face Lower Depth", "En Face Upper Depth": Value Change; User Event {
        n106 = event-data() -> ()  [unwired: 1 in, 2 out]
        n107 = for {
          tunnel: [w182] -> w181 mode=indexing
          tunnel: w180 -> [w183] mode=indexing
          n108 = property on="En Face Upper Depth" class="DigNum (strict)"() -> ("Value"=w187:i32)  [unwired: 2 in, 2 out]
          n109 = property on="En Face Lower Depth" class="DigNum (strict)"() -> ("Value"=w186:i32)  [unwired: 2 in, 2 out]
          n110 = for {
            N -> [w192]
            tunnel: w183 -> [w195] mode=indexing
            tunnel: w187 -> [w188]
            tunnel: w186 -> [w189]
            tunnel: [w193] -> w185 mode=indexing
            tunnel: [w192] -> w184
            n111 = Subtract(x=w189, y=w188) -> (x-y=w190:i32)
            n112 = Array Subset(array=w195, index=w188, length=w190) -> (w194:sgl[])
            n113 = To Single Precision Float(number=w194) -> (single precision float=w191:sgl[])
            n114 = Add Array Elements(numeric array=w191) -> (sum=w193:sgl)
          }
          n115 = Divide(x=w185, y=w184) -> (x/y=w182:sgl[])
        }
        "En Face" <- w181
      }
      event User Event {
        n116 = event-data() -> ()  [unwired: 1 in, 3 out]
        n117 = local read "A-Scans Per BScan"() -> (w202:i32)
        n118 = local read "Points Per A Scan"() -> (w203:i32)
        n119 = local read "Binary File Handle"() -> (w210:refnum<file>)
        n120 = property on="B-Scan Select" class="Slide (strict)"() -> ("Scale.Maximum"=w209:dbl)  [unwired: 2 in, 2 out]
        n121 = for {
          N: w209 -> [_]
          tunnel: w210 -> [w221]
          tunnel: [w214] -> w204 mode=indexing
          tunnel: w202 -> [w218]
          tunnel: w203 -> [w215]
          shift-right: [w219] -> w196
          shift-left: w207 -> [w219]
          i -> [w220]
          (unwired) FALSE ("Linear?")
          (unwired) u16 16 ("Card Resolution (bits)")
          n122 = local write "B-Scan Select"(w220) -> ()
          n123 = call "Read BScan.vi"("Points Per A Scan"=w215, "A-Scans Per BScan"=w218, "B-Scan"=w220, "Byte Stream File in"=w221) -> ("Array"=w213:u16[][])  [unwired: 7 in]
          n124 = for {
            shift-right: _ -> [_]
            shift-left: _ -> [_]
            tunnel: w213 -> [_] mode=indexing
            tunnel: [_] -> w212
          }
          n125 = local read "Bits"() -> (w217:dbl)
          n126 = local read "Range"() -> (w216:dbl)
          n127 = call "Labview_FFT.vi"("Channel A"=w212, "Range"=w216, "Bits"=w217) -> ("Int B-Scan Channel A"=w214:sgl[][])  [unwired: 12 in]
        }
        n128 = Generate User Event(user event=w208, event data cluster=FALSE ("event data"), error in=w196) -> (error out=w206:errorcluster)  [unwired: 1 in, 1 out]
        n129 = property on="B-Scan Select" class="Slide (strict)"(error in=w206, "Val(Sgnl)"=0 ("Value (Signaling)")) -> (error out=w201:errorcluster)  [unwired: 1 in, 1 out]
        n130 = property on="BScan" class="IntGraph (strict)"(error in=w201, "Cursor.Cursor Y"=50.0 ("Cursor.Cursor Position:Cursor Y")) -> (error out=w200:errorcluster)  [unwired: 1 in, 1 out]
        n131 = property on="BScan" class="IntGraph (strict)"(error in=w200, "Cursor.Cursor Y"=100.0 ("Cursor.Cursor Position:Cursor Y")) -> (error out=w199:errorcluster)  [unwired: 1 in, 1 out]
      }
      event "BScan": Cursor Release {
        # "First 2 cursors are the En Face slider, 3rd cursor is the A-Scan Selecter"
        n132 = event-data() -> ("CursIdx"=w226:i32)  [unwired: 1 in, 8 out]
        n133 = property on="BScan" class="IntGraph (strict)"() -> ("CrsrLis"=w229:T4)  [unwired: 2 in, 2 out]
        n134 = for {
          tunnel: w229 -> [w237] mode=indexing
          tunnel: [w236] -> w225 mode=indexing
          tunnel: [w235] -> w223 mode=indexing
          n135 = Unbundle By Name(w237) -> ("Position.Y"=w236:dbl, "Position.X"=w235:dbl)
        }
        n136 = Split 1D Array(array=w225, index=2) -> (first subarray=w227:dbl[])  [unwired: 1 out]
        n137 = Index Array(array=w223, index=2) -> (element=w222:dbl)
        n138 = case shown="0, 1, Default" w226 {
          tunnel: w227 -> [_ w232]
          tunnel: w222 -> [w231 _]
          frame 2 {
            n139 = property on="A-Scan Change" class="DigNum (strict)"("Val(Sgnl)"=w231) -> ()  [unwired: 2 in, 2 out]
          }
          frame 0, 1, Default {
            n140 = Array Max & Min(array=w232) -> (max value=w233:dbl, min value=w234:dbl)  [unwired: 2 out]
            n141 = property on="En Face Lower Depth" class="DigNum (strict)"("Val(Sgnl)"=w233) -> ()  [unwired: 2 in, 2 out]
            n142 = property on="En Face Upper Depth" class="DigNum (strict)"("Val(Sgnl)"=w234) -> ()  [unwired: 2 in, 2 out]
          }
        }
      }
      event "Min / Max in dB (Contrast)": Value Change {
        n143 = event-data() -> ("NewVal"=w245:cluster{dbl, dbl})  [unwired: 1 in, 5 out]
        n144 = Unbundle(w245) -> (w243:dbl, w244:dbl)
        n145 = Build Array(w243, w244) -> (w242:dbl[])
        n146 = Array Max & Min(array=w242) -> (max value=w240:dbl, min value=w241:dbl)  [unwired: 2 out]
        n147 = local write "Max"(w240) -> ()
        n148 = local write "Min"(w241) -> ()
        n149 = local read "B-Scan Select"() -> (w239:i32)
        n150 = property on="B-Scan Select" class="Slide (strict)"("Val(Sgnl)"=w239) -> ()  [unwired: 2 in, 2 out]
      }
      event Panel Close {
        n151 = event-data() -> ("VIRef"=w250:refnum<vi>)  [unwired: 1 in, 3 out]
        n152 = local read "Binary File Handle"() -> (w248:refnum<file>)
        n153 = Close File(refnum=w248) -> (error out=w247:errorcluster)  [unwired: 1 in, 1 out]
        n154 = call <vilib>:"Clear Errors.vi"("error in (no error)"=w247) -> ("error out"=w246:errorcluster)  [unwired: 5 in, 1 out]
        n155 = invoke class="VI" method="Abort VI"(reference=w250, error in=w246) -> ()  [unwired: 1 in, 3 out]
      }
      event "A-Scan Change": Value Change {
        n156 = event-data() -> ("NewVal"=w255:i32)  [unwired: 1 in, 5 out]
        n157 = local read "A-Scans Per BScan"() -> (w260:i32)
        n158 = local read "Binary File Handle"() -> (w261:refnum<file>)
        n159 = local read "Points Per A Scan"() -> (w259:i32)
        n160 = local read "B-Scan Select"() -> (w256:i32)
        n161 = call "Read BScan.vi"("Points Per A Scan"=w259, "A-Scans Per BScan"=w260, "B-Scan"=w256, "Byte Stream File in"=w261) -> ("Array"=w258:u16[][])  [unwired: 7 in]
        n162 = Index Array(array=w257, index (dim 0)=w256, index (dim 1)=w255) -> (element=w253:sgl[])  [unwired: 1 in]
        n163 = Index Array(array=w258, index (row)=w255) -> (element=w254:u16[])  [unwired: 1 in]
        n164 = flat-sequence {
          tunnel: w253 -> [w265]
          tunnel: w254 -> [w266]
          tunnel: [w266] -> w252
          tunnel: [w265] -> w251
          tunnel: w252 -> [w268]
          tunnel: w251 -> [w267]
          frame #0 {
            n165 = vi-ref "Processing.lvclass:View A-Scan.vi"() -> (w262:refnum<vi>)
            n166 = invoke class="VI" method="FP.Open"(reference=w262, "Activate"=TRUE ("Activate?"), "State"=T1."Standard") -> ()  [unwired: 2 in, 5 out]
          }
          frame #1 {
            n167 = call "View A-Scan.vi"("A-Scan Processed"=w267, "A-Scan (Raw)"=w268) -> ()  [unwired: 10 in]
          }
        }
      }
    }
  }
  "error out" <- w4
